vi "getLHeLevel.vi"(8 "error in (no error)":errorcluster, 11 "Instrument.Cryostat in":refnum<class "Instrument.Cryostat.lvclass">) -> (0 "error out":errorcluster, 2 "LHe Level (%)":dbl, 3 "Instrument.Cryostat out":refnum<class "Instrument.Cryostat.lvclass">)   [LabVIEW 2019, in "Instrument.Cryostat.lvclass"]
uses:
  Instrument.Cryostat.lvclass
  7bd3d363-2ea8-42d1-9339-e22a2a06b78c.vi
  Typedefs/Cryostat.commands--enum.ctl
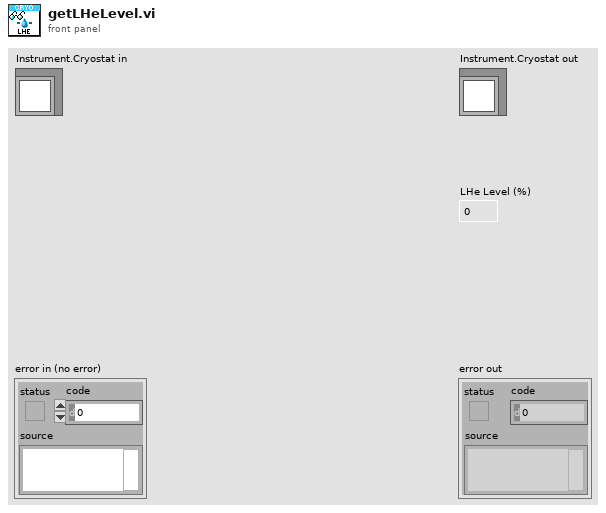
[diagram p1: front panel]
types:
  T1 = typedef "Instrument.Cryostat.lvclass/Cryostat.commands--enum.ctl" = enum16{"getLN2Level", "getLHeLevel", "getMagnet", "getMagnetVector", "setMagnet", "setMagnetVector", "getAngle", "setAngle", "getTemperature", "setTemperature", "getHeater", "setHeater", "getChamber", "setChamber", ""}
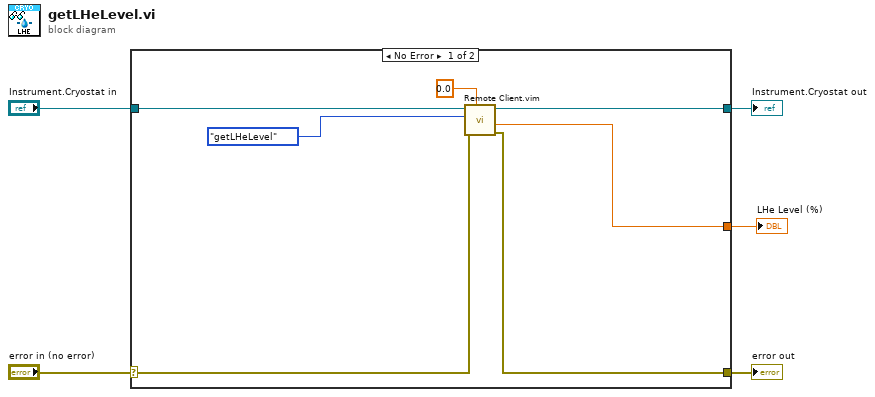
[diagram p0: block diagram]
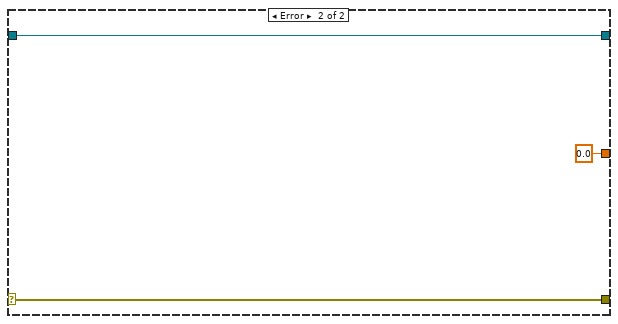
[diagram p2: hidden frame]
diagram:
  n1 = case shown="No Error" "error in (no error)" {
    selector: "error in (no error)" -> [w6 w15]
    tunnel: [w10 w15] -> w4
    tunnel: [w12 w14] -> w2
    tunnel: "Instrument.Cryostat in" -> [w8 w14]
    tunnel: [w11 0.0 ("Data out")] -> w1
    frame No Error {
      n2 = call "Remote Client.vim"("Data Out type"=0.0, "error in (no error)"=w6, "Command in"=Cryostat.commands--enum."getLHeLevel" ("commands"), "Instrument in"=w8) -> ("error out"=w10:errorcluster, "Data out"=w11:dbl, "Instrument out"=w12:refnum<class "Instrument.Cryostat.lvclass">)  [unwired: 4 in, 1 out]
    }
    frame Error {
    }
  }
  "error out" <- w4
  "Instrument.Cryostat out" <- w2
  "LHe Level (%)" <- w1
